vi "Reverse Find.vi"(7 "Character":string, 11 "String":string) -> (3 "Position":i32)   [LabVIEW 2018, in "Toolkit.lvlib" / "Lexer.lvclass"]
uses:
  Lexer.lvclass
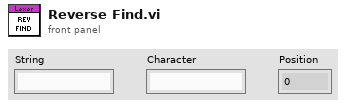
[diagram p1: front panel]
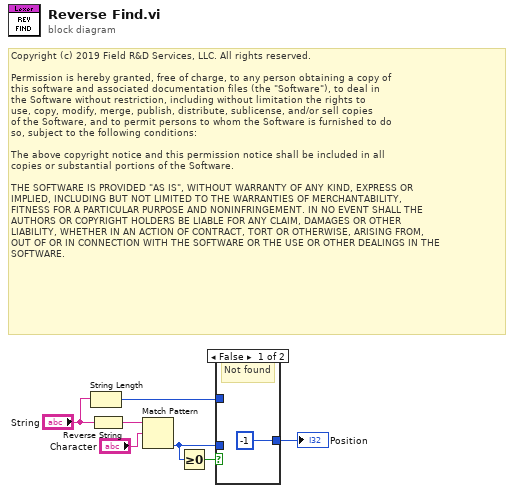
[diagram p0: block diagram]
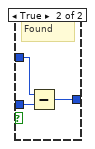
[diagram p2: hidden frame]
diagram:
  # "Copyright (c) 2019 Field R&D Services, LLC. All rights reserved.\n\nPermission is hereby granted, free of charge, to any person obtaining a copy of\nthis software and associated documentation files (the \"Software\"), to deal in\nthe Software without restriction, including without limitation the rights to\nuse, copy, modify, merge, publish, distribute, sublicense, and/or sell copies\nof the Software, and to permit persons to whom the Software is furnished to do\nso, subject to the following conditions:\n\nThe above copyright notice and this permission notice shall be included in all\ncopies or substantial portions of the Software.\n\nTHE SOFTWARE IS PROVIDED \"AS IS\", WITHOUT WARRANTY OF ANY KIND, EXPRESS OR\nIMPLIED, INCLUDING BUT NOT LIMITED TO THE WARRANTIES OF MERCHANTABILITY,\nFITNESS FOR A PARTICULAR PURPOSE AND NONINFRINGEMENT. IN NO EVENT SHALL THE\nAUTHORS OR COPYRIGHT HOLDERS BE LIABLE FOR ANY CLAIM, DAMAGES OR OTHER\nLIABILITY, WHETHER IN AN ACTION OF CONTRACT, TORT OR OTHERWISE, ARISING FROM,\nOUT OF OR IN CONNECTION WITH THE SOFTWARE OR THE USE OR OTHER DEALINGS IN THE\nSOFTWARE."
  n1 = String Length(string="String") -> (length=w3:i32)
  n2 = Reverse String(1:"String") -> (0:w2:string)
  n3 = Match Pattern(string=w2, regular expression="Character") -> (offset past match=w6:i32)  [unwired: 1 in, 3 out]
  n4 = Greater Or Equal To 0?(x=w6) -> (x >= 0?=w4:bool)
  n5 = case shown="False" w4 {
    tunnel: w3 -> [_ w11]
    tunnel: w6 -> [_ w10]
    tunnel: [-1 w9] -> w7
    frame False {
      # "Not found"
    }
    frame True {
      # "Found"
      n6 = Subtract(x=w11, y=w10) -> (x-y=w9:i32)
    }
  }
  "Position" <- w7
